vi "Group Data and Triggers for Display 20221121.vi"(9 "scaling coefficients":T3[](array[typedef]), 10 "TrigCfg 0":T2, 11 "Data waveform":T1(array[cluster])) -> (3 "Data for Display":T1(array[cluster]))   [LabVIEW 2021]
doc: "Sort and group Acquisition Data and thresholds. This preps for chart display.\n\nNote that this only works with one channel."
uses:
  <instrlib>/_niInstr/Multirecord Acquisition/Interface/v1/Host/Public/Scaling Coefficient.ctl
  <instrlib>/_niInstr/Multirecord Acquisition/Interface/v1/Host/niInstr Multirecord Acquisition v1 Host.lvclass
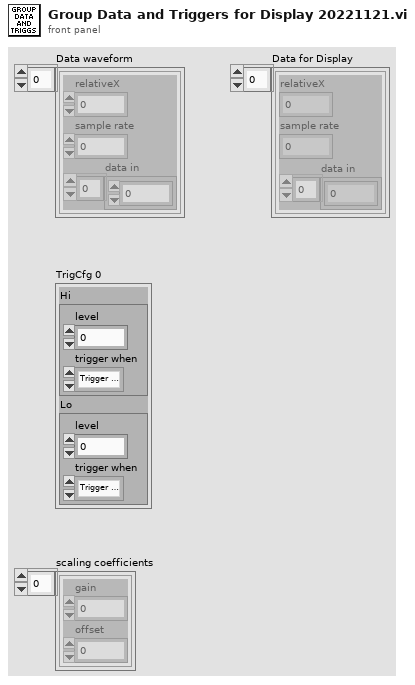
[diagram p1: front panel]
types:
  T1 = cluster{"relativeX":dbl, "sample rate":dbl, "data in":dbl[]}[]
  T2 = cluster{"Hi":cluster{"level":fxp<+/-,18,1>, "trigger when":enum8{"Trigger Above", "Trigger Below"}}, "Lo":cluster{"level":fxp<+/-,18,1>, "trigger when":enum8{"Trigger Above", "Trigger Below"}}}
  T3 = typedef "niInstr Multirecord Acquisition v1 Host.lvclass/Scaling Coefficient.ctl" = cluster{"gain":dbl, "offset":dbl}
  T4 = cluster{"relativeX":dbl, "sample rate":dbl, "data in":dbl[]}
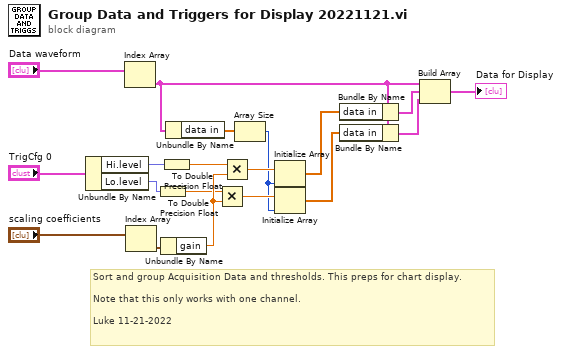
[diagram p0: block diagram]
diagram:
  # "Sort and group Acquisition Data and thresholds. This preps for chart display.\n\nNote that this only works with one channel.\n\nLuke 11-21-2022"
  n1 = Unbundle By Name("TrigCfg 0") -> ("Hi.level"=w6:fxp<+/-,18,1>, "Lo.level"=w9:fxp<+/-,18,1>)
  n2 = Index Array(array="Data waveform") -> (element=w7:T4)  [unwired: 1 in]
  n3 = Index Array(array="scaling coefficients") -> (element=w16:T3)  [unwired: 1 in]
  n4 = To Double Precision Float(number=w9) -> (double precision float=w12:dbl)
  n5 = Unbundle By Name(w16) -> ("gain"=w19:dbl)
  n6 = To Double Precision Float(number=w6) -> (double precision float=w11:dbl)
  n7 = Unbundle By Name(w7) -> ("data in"=w8:dbl[])
  n8 = Multiply(x=w12, y=w19) -> (x*y=w18:dbl)
  n9 = Multiply(x=w11, y=w19) -> (x*y=w17:dbl)
  n10 = Array Size(array=w8) -> (size(s)=w10:i32)
  n11 = Initialize Array(w17, w10) -> (w13:dbl[])
  n12 = Initialize Array(w18, w10) -> (w14:dbl[])
  n13 = Bundle By Name(cluster=w7, "data in"=w13) -> (w2:T4)
  n14 = Bundle By Name(cluster=w7, "data in"=w14) -> (w3:T4)
  n15 = Build Array(w7, w2, w3) -> (→"Data for Display":T1)
